vi "NI-USB6001.vi"() -> ()   [LabVIEW 2020]
uses:
  <vilib>/Utility/miscctls.llb/LVPointTypeDef.ctl
  LabVIEW 2020 Toolkits/toolkits_lv2020_32bit/Synchronization.llb/SynchRefs_SetGet.ctl
  LabVIEW 2020 Toolkits/VI Server Toolkit/VI Server Libraries/VI Server_GetControl.llb/VI Server_STR_Get.vi
  LabVIEW 2020 Toolkits/VI Server Toolkit/VI Server Libraries/VI Server_Set Controls.llb/Set STR Control.vi
  LabVIEW 2020 Toolkits/VI Server Toolkit/VI Server Libraries/VI Server_GetControl.llb/VI Server_DBL_Get.vi
  LabVIEW 2020 Toolkits/VI Server Toolkit/VI Server Libraries/VI Server_GetControl.llb/VI Server_Slide_DBL_Get.vi
  LabVIEW 2020 Toolkits/VI Server Toolkit/VI Server Libraries/VI Server_GetControl.llb/VI Server_DAQmx_Device_Get.vi
  LabVIEW 2020 Toolkits/VI Server Toolkit/VI Server Toolkit LV2013.lvlib
panel:
  in  "LastAction.AddToSecuence":bool
  out "System.Message":string="Instrument Initialization Successful." caption="System Message"
  in  "Help":bool
  in  "FP.Hide":bool caption="FrontPanel.Hide"
  in  "EXIT":bool
  in  "Tab.Main":T1(tab)
  in  "AI.Graph.Plots":u16(ring) items=["NI-USB6001/ai0"]
  in  "AI.MultiChannelAcquisition":bool
  in  "AI.PhysicalChannel.Include":bool
  out "AI.ActualSampleRate":dbl=1000.0 caption="Actual Sample Rate" format="%0.2f"
  out "AI.WaveformGraph":waveform(dbl)[](graph) caption="Waveform Graph"
  out "AI.Averaged.Mesurement":dbl caption="Averaged Mesurement" format="%0.4f V"
  in  "AI.Measure":bool
  in  "AI.Number.Of.Samples":i32=100 caption="Number Of Samples"
  in  "AI.SampleRate":dbl=1000.0 caption="Sample Rate" format="%0.0f Hz"
  in  "AI.MinInputLimit":dbl caption="Min Input Limit" min=-10.0 max=10.0 format="%0.3f V"
  in  "AI.MaxInputLimit":dbl caption="Max Input Limit" min=-10.0 max=10.0 format="%0.3f V"
  in  "AI.TerminalConfiguration":u16(ring)=65535 caption="Terminal Configuration" items=["default"=65535, "RSE"=10083, "NRSE"=10078, "Differential"=10106, "Pseudodifferential"=12529]
  in  "AI.Sample.Mode":u16(ring)=12522 caption="Sample Mode" items=["Finite Samples"=10178, "Continuous Samples"=10123]
  in  "AI.Physical.Channel":tag="Dev1/ai0" caption="Physical Channel"
  in  "AO.Update":bool
  out "AO.WaveformGraph":waveform(dbl)(graph) caption="Waveform Graph"
  in  "AO.SampleMode":u16(ring) caption="Sample Mode" items=["Finite Samples"=10178, "Continious Samples"=10123, "Hardware Timed Single Point"=12522]
  in  "AO.OutputVoltage":dbl(slide) caption="Output Voltage" scale=-10.0..10.0 scale format="%0.3f V"
  in  "AO.SinewaveFrequency":dbl=5.0 caption="Sinewave Frequency" min=1e-36 max=5.0 format="%0.2p Hz"
  in  "AO.GenerationMode":u16(ring) caption="Generation Mode" items=["Voltage DC", "Voltage Sine Wave Generation"]
  in  "AO.NumberOfSamples":i32=1000 caption="Number Of Samples" min=2
  in  "AO.SampleRate":dbl=5000.0 caption="Sample Rate" min=1e-07 max=5000.0
  in  "AO.Sample.Clock.Source":tag="OnboardClock" caption="Sample Clock Source"
  out "AO.ActualSampleRate":dbl=1000.0 caption="Actual Sample Rate" format="%0.2f"
  in  "AO.MaxVoltage":dbl=5.0 caption="Max Voltage" format="%0.3f V"
  in  "AO.MinVoltage":dbl=-5.0 caption="Min Voltage" format="%0.3f V"
  in  "AO.Physical.Channel":tag="Dev1/ai0" caption="Physical Channel"
  in  "AO.Output":bool
  out "DO.Port.State.Verify":bool caption="Verified"
  out "DO.Line.State.Verify":bool caption="Verified"
  in  "DO.Line.State":bool caption="State"
  in  "DO.Line":tag="Dev1/port0/line0:7" caption="Line"
  in  "DO.Line.Update":bool caption="Update:"
  in  "DO.Port.Update":bool
  in  "DO.Port.Lines.7:0":u8 caption="Port&Lines 7:0" format="%08b"
  in  "DO.Port":tag="Dev1/port0/line0:7" caption="Port"
  out "DI.Line.State":bool caption="State"
  in  "DI.Port.Update":bool
  out "DI.Port.Lines.0:7":u8 caption="Port&Lines 7:0" format="%08b"
  in  "DI.Port":tag="Dev1/port0/line0:7" caption="Port"
  in  "DI.Line":tag="Dev1/port0/line0:7" caption="Line"
  in  "DI.Line.Update":bool caption="Update:"
  out "ctr0.In.Count":u32 caption="Counts:"
  in  "Cntr.In.Start":bool
  in  "Cntr.In.IntegrationTime":u32=10 format="%.0f msec"
  in  "Cntr.In.Sample.Clock.Source":tag="PFI0" caption="Sample Clock Source"
  in  "Cntr.In.ActiveEdge":u16(ring)=10280 caption="Active Edge" items=["Rising"=10280, "Falling"=10171]
  in  "Cntr.In.Input.Terminal":tag="OnboardClock" caption="Input.Terminal"
  in  "Cntr.In.Channel":tag="Dev1/port0/line0:7" caption="Channel Name"
  in  "TestCase.Execute.All":bool
  in  "TestCase.Execute.Selected":bool
  out "TestCase.SAVE.Success":bool
  in  "TestCase.SAVE":bool
  in  "SequenceFile.Open":bool
  in  "SequenceFile":path caption="Secuence File"
  in  "TestCase.Execute.Step.Pause":bool
  in  "TestCase.Execute.Steps":u16(ring) caption="Test Case: Pause Before Step" items=["1", "2", "3", "4", "5", "6", "7", "8", "9", "10"]
  in  "TestCase.Execute.ABORT":bool
  in  "TestCase.Execute.Next":bool
  in  "TestCase.Execute.Pause":bool
  out "TestCase.ExecutionTime":dbl caption="Execution Time:" format="%0.3f sec"
  in  "TestCase.Execution.StepTime":u32 caption="Seq. Execution: Step Time" format="%d msec"
  in  "TestCaseConfiguration":i32[](listbox) caption="Test Case Configuration"
  in  "TestCase.StepDescription":string caption="Step Description:"
  in  "ProductType":string="USB-6343 (BNC)" caption="Product Type"
  in  "VI.WindowsTitle":string caption="Windows Title"
  in  "DAQmx.Device":tag caption="DAQmx: Device"
  in  "Cont.Measurements.CycleTime":u32 caption="Continius Measurements:\nCycleTime"
  in  "UDP.Test.String2.Send":bool
  in  "UDP.Test.String2":string caption="UDP: Test String 2"
  in  "UDP.Port.BC":u16=58433 caption="UDP: Port.BC"
  in  "UDP.Port.RT":u16=58432 caption="UDP: Port.RT"
  in  "UDP.LocalPort.Write":u16=58434 caption="UDP: Local Port.Write"
  in  "UDP.IP.Address":string="234.5.6.7" caption="UDP: IP Address"
  in  "UDP.Test.String1.Send":bool
  in  "UDP.Test.String1":string caption="UDP: Test String 1"
  in  "UDP.Responce.String.Monitor":bool
  out "UDP.ExecEng.Message.String":string caption="UDP: Execution Engine Message String"
  out "error out":errorcluster={"status"=TRUE, "code"=1055, "source"="Property Node in VI Server Toolkit LV2013.lvlib:VI server_Set Control Value from String Format.vi:5200001->DMM6500_UDP_ExecEng_Instruction_APPLY.vi->DMM6500_UDP_MAIN.vi->Keithley2100.vi"}
  in  "error in":errorcluster
  # "Important Note: Analog Input configuration shall\nstart from Physical Channel selection!"
  # "Digital Input"
  # "Digital Output"
  # "Onboard Clock is not supported as an \nInput Terminal for counter measurements."
  # "Counter Input"
  # "Counter Input"
  # "M"
  # "Multicast IP addresses must be in the 224.0.0.0 to 239.255.255.255 range."
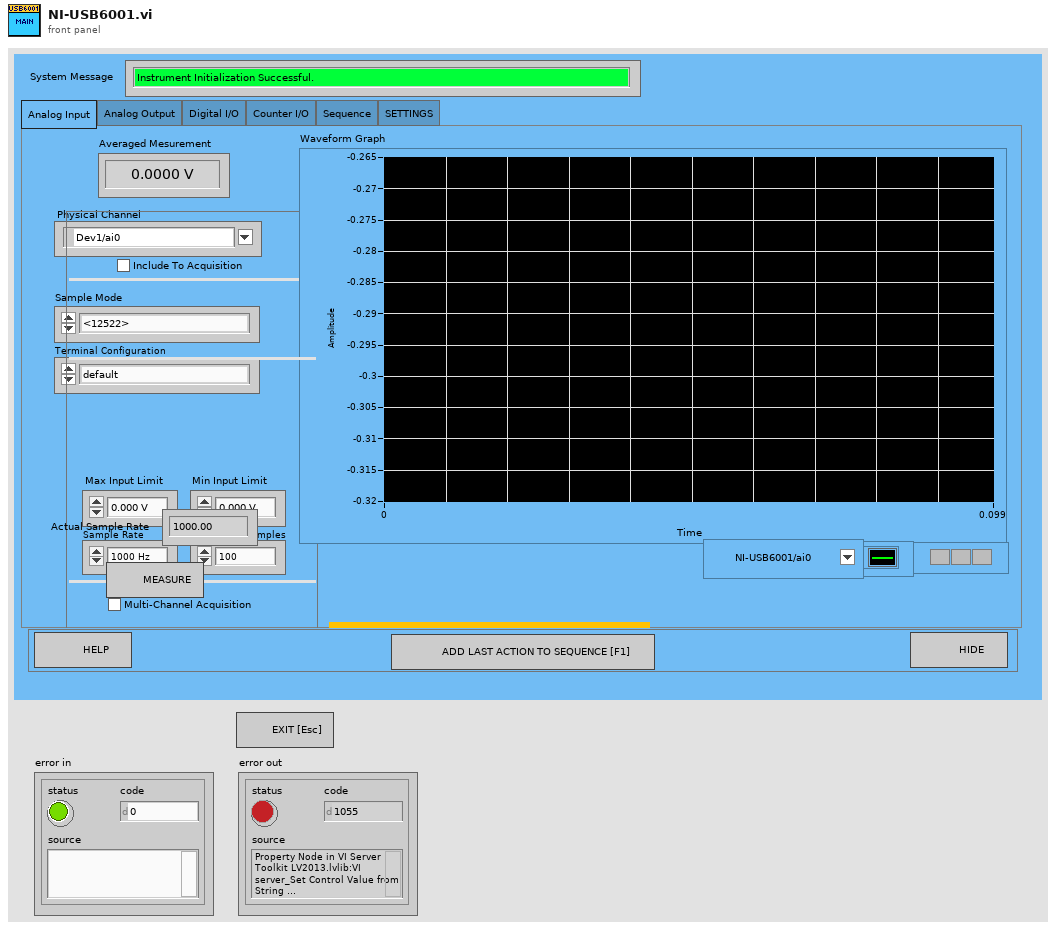
[diagram p1: front panel]
types:
  T1 = enum32{"Analog Input", "Analog Output", "Digital I/O", "Counter I/O", "Sequence", "SETTINGS"}
  T2 = typedef "LVPointTypeDef.ctl" = cluster{"Horizontal":i16, "Vertical":i16}
  T3 = typedef "VI Server_RefsCluster.ctl" = cluster{"Labels":string[], "Refs":refnum<vi>[], "VI Ref":refnum<vi>}
  T4 = typedef "SynchRefs_SetGet.ctl" = enum16{"Set", "Get"}
  T5 = cluster{"Color":u32, "PointStyle":u8, "LineStyle":u8, "Interp":u8, "LineWidth":u8, "BarPlotStyle":u8, "FillTo":i16, "XScaleIdx":u32, "YScaleIdx":u32, "Anti-Aliased":bool, "LabelFormat":u8, "TransitionType":u8, "TransitionLocation":u8, "DigitalLineStyle":u8}
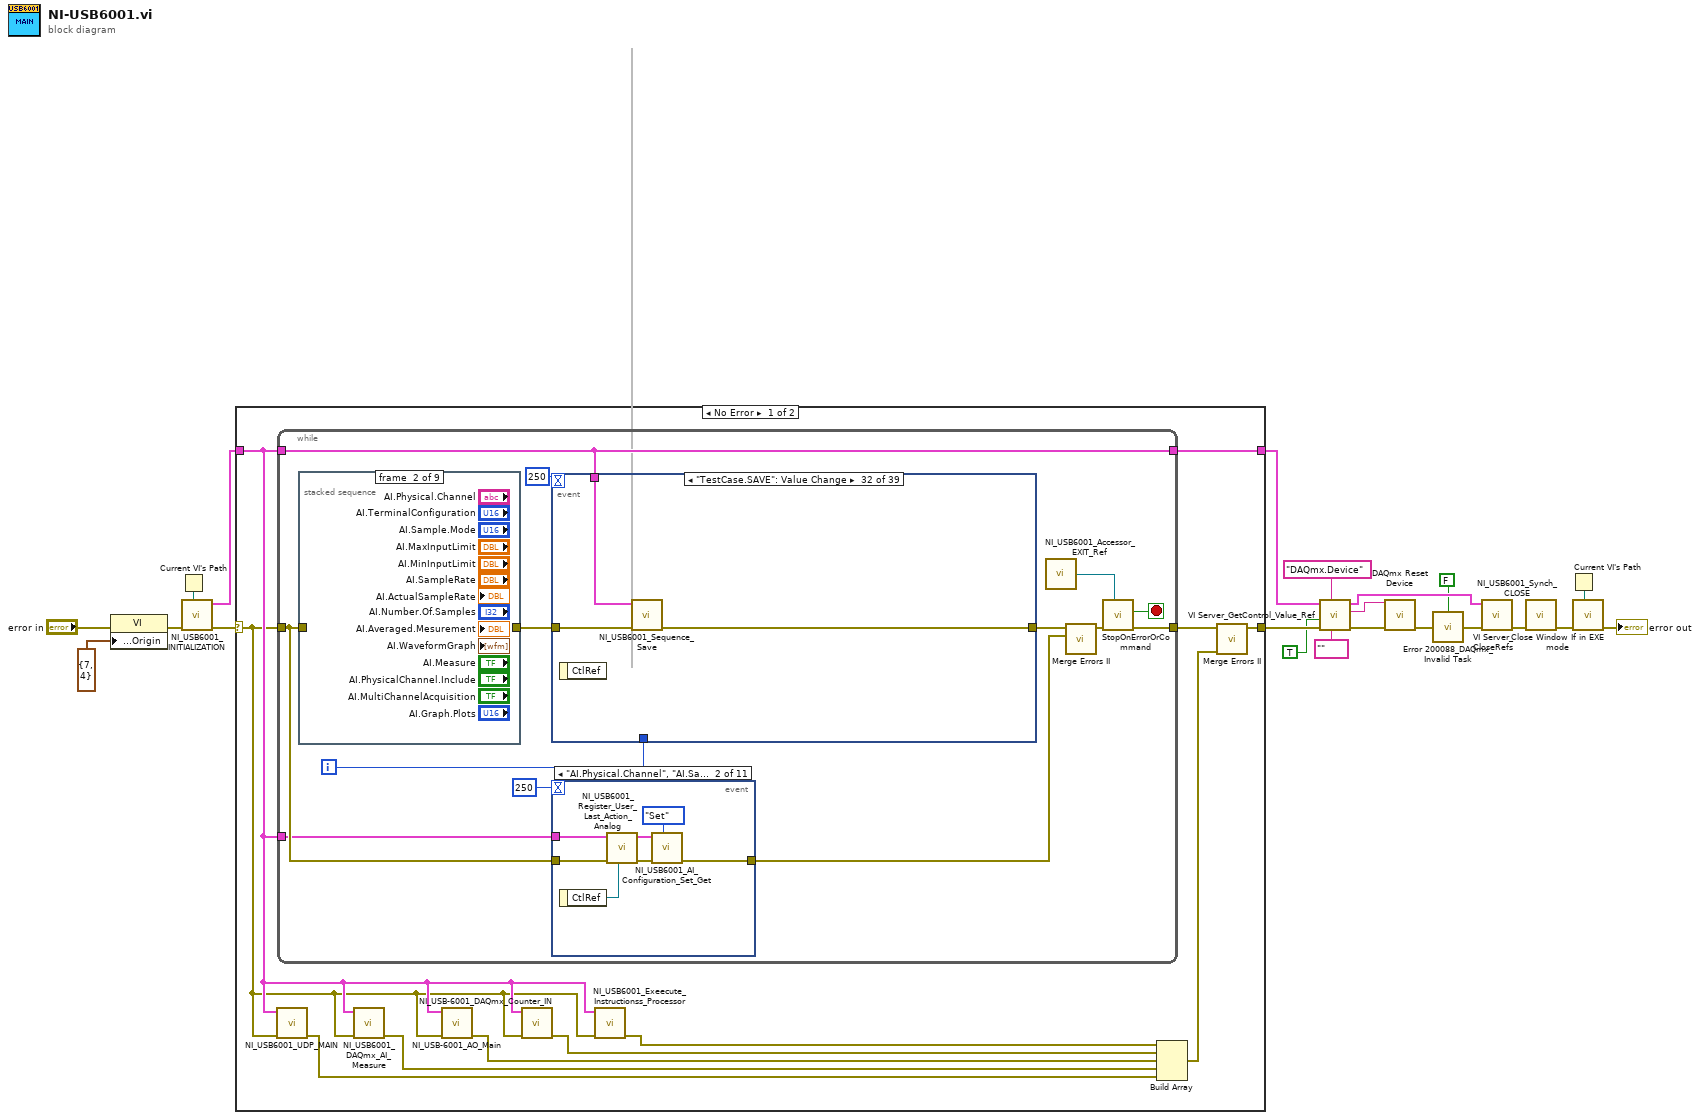
[diagram p0: block diagram]
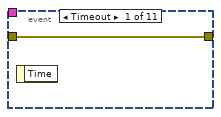
[diagram p2: hidden frame]
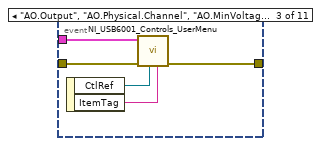
[diagram p3: hidden frame]
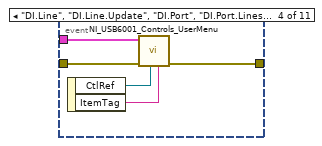
[diagram p4: hidden frame]
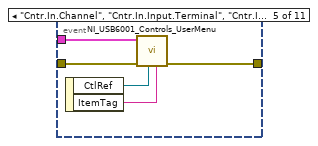
[diagram p5: hidden frame]
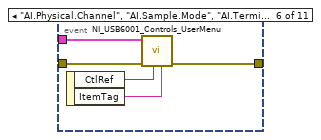
[diagram p6: hidden frame]
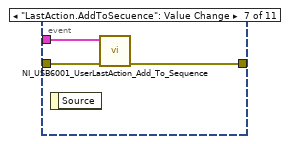
[diagram p7: hidden frame]
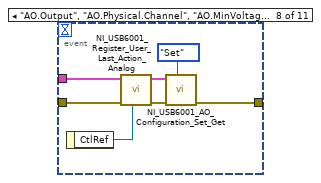
[diagram p8: hidden frame]
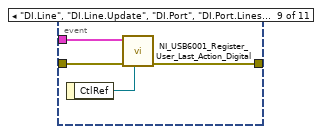
[diagram p9: hidden frame]
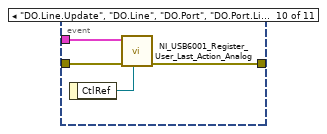
[diagram p10: hidden frame]
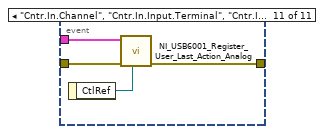
[diagram p11: hidden frame]
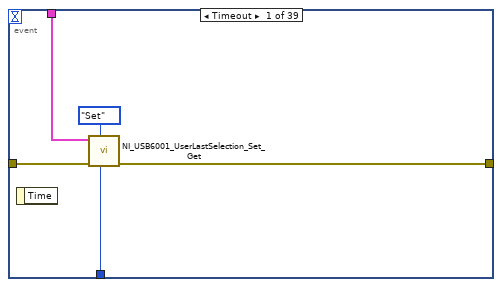
[diagram p12: hidden frame]
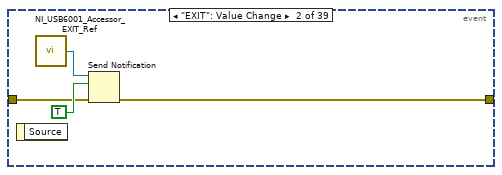
[diagram p13: hidden frame]
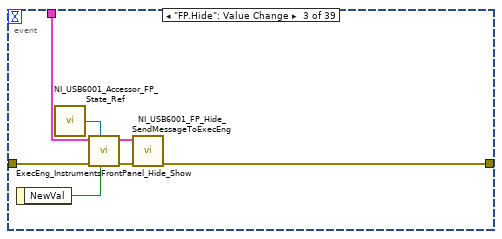
[diagram p14: hidden frame]
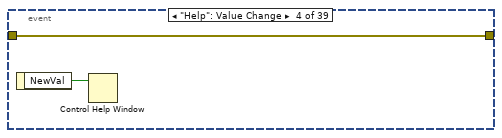
[diagram p15: hidden frame]
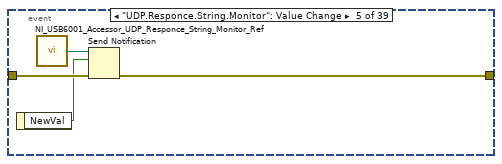
[diagram p16: hidden frame]
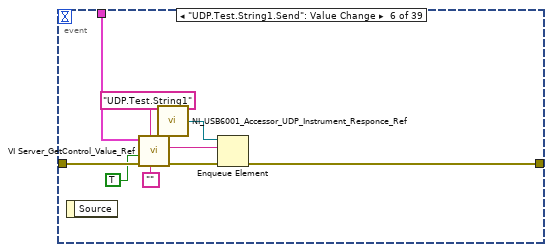
[diagram p17: hidden frame]
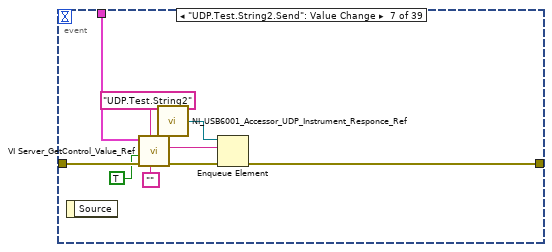
[diagram p18: hidden frame]
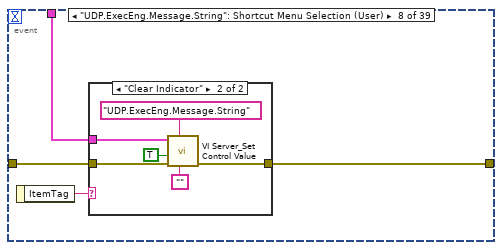
[diagram p19: hidden frame]
diagram:
  n1 = property class="VI"(error in="error in", "Front Panel Window:Origin"=T2 {"Horizontal"=7, "Vertical"=4}) -> (error out=w21:errorcluster)  [unwired: 1 in, 1 out]
  n2 = Current VI's Path() -> (path=w1:path)
  n3 = call "NI_USB6001_INITIALIZATION.vi"("Top VI Path"=w1, "error in (no error)"=w21) -> ("error out"=w20:errorcluster, "VI Server Cluster.OUT"=w19:T3)  [unwired: 8 in]
  n4 = case shown="No Error" w20 {
    selector: w20 -> [w23 w321]
    tunnel: [w29 w321] -> w12
    tunnel: w19 -> [w24 w320]
    tunnel: [w32 w320] -> w10
    frame No Error {
      n5 = call "NI_USB6001_UDP_MAIN.vi"("error in (no error)"=w23, "VI Server.RefsCluster"=w24) -> ("error out"=w31:errorcluster)  [unwired: 9 in]
      n6 = while {
        tunnel: w23 -> [w37]
        tunnel: [w41] -> w30
        tunnel: w24 -> [w42]
        tunnel: [w42] -> w32
        tunnel: w24 -> [w36]
        i -> [w43]
        stop <- w40 stop-if-true
        n7 = stacked-sequence {
          tunnel: w37 -> [w319 _ _ _ _ _ _ _ _]
          tunnel: [w319 _ _ _ _ _ _ _ _] -> w45
          frame #0 {
          }
          frame #1 {
          }
          frame #2 {
          }
          frame #3 {
          }
          frame #4 {
          }
          frame #5 {
          }
          frame #6 {
          }
          frame #7 {
          }
          frame #8 {
          }
        }
        n8 = event shown="[31] \"TestCase.SAVE\": Value Change" {
          selector: _ -> [_ _ _ _ _ _ _ _ _ _ _ _ _ _ _ _ _ _ _ _ _ _ _ _ _ _ _ _ _ _ _ _ _ _ _ _ _ _ _]
          dyn-events: _ -> [_ _ _ _ _ _ _ _ _ _ _ _ _ _ _ _ _ _ _ _ _ _ _ _ _ _ _ _ _ _ _ _ _ _ _ _ _ _ _]
          timeout: 250 -> [_ _ _ _ _ _ _ _ _ _ _ _ _ _ _ _ _ _ _ _ _ _ _ _ _ _ _ _ _ _ _ _ _ _ _ _ _ _ _]
          tunnel: w45 -> [w99 w101 w110 w113 w117 w126 w135 w139 w152 w158 w171 w174 w175 w180 w183 w190 w194 w198 w204 w212 w237 w240 w244 w247 w250 w253 w257 w266 w274 w277 w282 w285 w288 w291 w294 w298 w310 w312 w316]
          tunnel: w43 -> [w98 _ _ _ _ _ _ _ _ _ _ _ _ _ _ _ _ _ _ _ _ _ _ _ _ _ _ _ _ _ _ _ _ _ _ _ _ _ _]
          tunnel: [w96 w103 w111 w113 w115 w124 w133 w137 w149 w154 w163 w172 w175 w176 w182 w186 w191 w197 w203 w206 w225 w239 w242 w245 w248 w252 w255 w263 w272 w278 w280 w283 w286 w289 w292 w297 w309 w314 w315] -> w35
          tunnel: w42 -> [w97 _ w107 _ _ w123 w132 w136 w151 w157 w170 w173 _ w179 w181 w189 w193 _ _ w211 w235 w238 w243 w246 w249 w254 w256 _ w273 w276 w281 w284 w287 w290 w293 w296 _ _ _]
          event Timeout {
            n9 = event-data() -> ()  [unwired: 1 in, 1 out]
            n10 = call "NI_USB6001_UserLastSelection_Set_Get.vi"("LoopCounter"=w98, "SynchRefs.Set/Get"=SynchRefs_SetGet."Set", "error in"=w99, "VI Server.RefsCluster"=w97) -> ("error out"=w96:errorcluster)  [unwired: 6 in, 1 out]
          }
          event "EXIT": Value Change {
            n11 = event-data() -> ()  [unwired: 1 in, 1 out]
            n12 = call "NI_USB6001_Accessor_EXIT_Ref.vi"() -> ("EXIT"=w104:refnum<notifier>)  [unwired: 6 in]
            n13 = Send Notification(notification=TRUE, notifier=w104, error in (no error)=w101) -> (error out=w103:errorcluster)  [unwired: 1 out]
          }
          event "FP.Hide": Value Change {
            n14 = event-data() -> ("NewVal"=w108:bool)  [unwired: 1 in]
            n15 = call "NI_USB6001_Accessor_FP_State_Ref.vi"() -> ("FP.State"=w105:refnum<notifier>)  [unwired: 6 in]
            n16 = call "ExecEng_InstrumentsFrontPanel_Hide_Show.vi"("FP.Hide/Show"=w108, "FP.State"=w105, "error in (no error)"=w110, "VI Server Cluster"=w107) -> ("error out"=w109:errorcluster, "VI Server Cluster DUP"=w106:T3)  [unwired: 6 in]
            n17 = call "NI_USB6001_FP_Hide_SendMessageToExecEng.vi"("error in (no error)"=w109, "VI Server Cluster"=w106) -> ("error out"=w111:errorcluster)  [unwired: 9 in]
          }
          event "Help": Value Change {
            n18 = event-data() -> ("NewVal"=w112:bool)  [unwired: 1 in]
            n19 = Control Help Window(1:w112) -> ()  [unwired: 1 in]
          }
          event "UDP.Responce.String.Monitor": Value Change {
            n20 = event-data() -> ("NewVal"=w114:bool)  [unwired: 1 in]
            n21 = call "NI_USB6001_Accessor_UDP_Responce_String_Monitor_Ref.vi"() -> ("UDP.ExecEng.Command.String.Monitor"=w116:refnum<notifier>)  [unwired: 6 in]
            n22 = Send Notification(notification=w114, notifier=w116, error in (no error)=w117) -> (error out=w115:errorcluster)  [unwired: 1 out]
          }
          event "UDP.Test.String1.Send": Value Change {
            n23 = event-data() -> ()  [unwired: 1 in, 1 out]
            n24 = call-poly "VI Server_GetControl_Value_Ref.vi"("DataType"="", "Control.Label"="UDP.Test.String1", "error in"=w126, "SingleInstance"=TRUE, "VI Server.RefsCluster"=w123) -> ("error out"=w125:errorcluster, "Value"=w118:string)  [unwired: 3 in, 2 out]
            n25 = call "NI_USB6001_Accessor_UDP_Instrument_Responce_Ref.vi"() -> ("UDP.Instrument.Responce.Q"=w119:refnum<queue>)  [unwired: 6 in]
            n26 = Enqueue Element(queue=w119, element=w118, error in (no error)=w125) -> (error out=w124:errorcluster)  [unwired: 1 in, 2 out]
          }
          event "UDP.Test.String2.Send": Value Change {
            n27 = event-data() -> ()  [unwired: 1 in, 1 out]
            n28 = call-poly "VI Server_GetControl_Value_Ref.vi"("DataType"="", "Control.Label"="UDP.Test.String2", "error in"=w135, "SingleInstance"=TRUE, "VI Server.RefsCluster"=w132) -> ("error out"=w134:errorcluster, "Value"=w127:string)  [unwired: 3 in, 2 out]
            n29 = call "NI_USB6001_Accessor_UDP_Instrument_Responce_Ref.vi"() -> ("UDP.Instrument.Responce.Q"=w128:refnum<queue>)  [unwired: 6 in]
            n30 = Enqueue Element(queue=w128, element=w127, error in (no error)=w134) -> (error out=w133:errorcluster)  [unwired: 1 in, 2 out]
          }
          event "UDP.ExecEng.Message.String": Shortcut Menu Selection (User) {
            n31 = event-data() -> ("ItemTag"=w138:string)  [unwired: 1 in]
            n32 = case shown="\"Clear Indicator\"" w138 {
              tunnel: w139 -> [w140 w146]
              tunnel: [w140 w145] -> w137
              tunnel: w136 -> [_ w144]
              frame "", Default {
              }
              frame "Clear Indicator" {
                n33 = call-poly "VI Server_Set Control Value.vi"("New Value"="", "Label"="UDP.ExecEng.Message.String" ("Control.Label"), "error in"=w146, "Single Instance (T)"=TRUE ("SingleInstance"), "VI Server Cluster"=w144) -> ("error out"=w145:errorcluster)  [unwired: 4 in, 2 out]
              }
            }
          }
          event "DAQmx.Device": Value Change {
            n34 = event-data() -> ("NewVal"=w148:tag)  [unwired: 1 in]
            n35 = call "NI_USB6001_DAQmx_LimitPhysicalChannelsToDevice.vi"("error in (no error)"=w152, "VI Server Cluster"=w151) -> ("error out"=w150:errorcluster, "VI Server Cluster.DUP"=w147:T3)  [unwired: 7 in, 1 out]
            n36 = call "NI_USB6001_DAQmx_DeviceName_Changed_UpdateSet_Get_Sections.vi"("DAQmx.Device"=w148, "error in (no error)"=w150, "VI Server Cluster"=w147) -> ("error out"=w149:errorcluster)  [unwired: 8 in]
          }
          event "AI.Physical.Channel": Value Change {
            n37 = event-data() -> ()  [unwired: 1 in, 1 out]
            n38 = call "NI_USB6001_AI_Configuration_Set_Get.vi"("SynchRefs.Set/Get"=SynchRefs_SetGet."Get", "error in (no error)"=w158, "VI Server Cluster"=w157) -> ("error out"=w153:errorcluster, "VI Server Cluster.DUP"=w155:T3)  [unwired: 6 in, 1 out]
            n39 = call "NI_USB6001_AI_Graph_PopulatePlotSelector.vi"("error in (no error)"=w153, "VI Server Cluster"=w155) -> ("error out"=w154:errorcluster)  [unwired: 9 in]
          }
          event "TestCaseConfiguration": Value Change {
            n40 = event-data() -> ()  [unwired: 1 in, 1 out]
            n41 = call "VI Server_M_ClmnListBox_1orMoreSelection_ItemNames_GET.vi"("Label"="TestCaseConfiguration", "error in"=w171, "SingleInstance"=TRUE, "VI Server.RefsCluster"=w170) -> ("error out"=w165:errorcluster, "Item Names"=w167:string[][], "VI Server.RefsCluster.DUP"=w164:T3, "Value"=w166:i32[])  [unwired: 1 in, 3 out]
            n42 = Index Array(array=w166) -> (element=w159:i32)  [unwired: 1 in]
            n43 = Index Array(array=w167, index (row)=w159, index (col)=0 ("index (row)")) -> (element=w160:string)
            n44 = call "VI Server_Set Text Ring by Item Selected_SignalingValue.vi"("Label"="TestCase.Execute.Steps" ("Control.Label"), "error in"=w165, "Item"=w160, "VI Server Cluster"=w164) -> ("error out"=w163:errorcluster)  [unwired: 5 in, 2 out]
          }
          event "AI.MultiChannelAcquisition": Value Change {
            n45 = event-data() -> ()  [unwired: 1 in, 1 out]
            n46 = call "NI_USB6001_AI_MultiChannelACQ_UpdateGraph_Plots.vi"("error in (no error)"=w174, "VI Server Cluster"=w173) -> ("error out"=w172:errorcluster)  [unwired: 9 in]
          }
          event "AI.Measure": Value Change {
            n47 = event-data() -> ()  [unwired: 1 in, 1 out]
          }
          event "AI.WaveformGraph": Plot Attribute Change {
            n48 = event-data() -> ("OldAttrib"=w178:T5, "NewAttrib"=w177:T5)  [unwired: 1 in]
            n49 = call "NI_USB6001_AI_Graph_PlotAttribute_ValueChanged.vi"("NewAttrib"=w177, "OldAttrib"=w178, "error in (no error)"=w180, "VI Server Cluster"=w179) -> ("error out"=w176:errorcluster)  [unwired: 7 in]
          }
          event "AO.Physical.Channel": Value Change {
            n50 = event-data() -> ()  [unwired: 1 in, 1 out]
            n51 = call "NI_USB6001_AO_Configuration_Set_Get.vi"("error in (no error)"=w183, "VI Server Cluster"=w181) -> ("error out"=w182:errorcluster)  [unwired: 7 in, 2 out]
          }
          event "AO.GenerationMode": Value Change {
            n52 = event-data() -> ("NewVal"=w184:u16)  [unwired: 1 in]
            n53 = call "NI_USB6001_AO_GenerationMode.vi"("AO.GenerationMode"=w184, "error in (no error)"=w190, "VI Server Cluster"=w189) -> ("error out"=w187:errorcluster)  [unwired: 7 in, 1 out]
            n54 = call "NI_USB-6001_Accessor_ao_Waveform_Array_Update_Ref.vi"() -> ("ao.Waveform.Array.Update"=w185:refnum<notifier>)  [unwired: 6 in]
            n55 = Send Notification(notification=TRUE, notifier=w185, error in (no error)=w187) -> (error out=w186:errorcluster)  [unwired: 1 out]
          }
          event "AO.OutputVoltage", "AO.SinewaveFrequency": Value Change {
            n56 = event-data() -> ()  [unwired: 1 in, 1 out]
            n57 = call "VI Server_CycleEventBySignalingValue.vi"("Label"="AO.GenerationMode", "error in"=w194, "VI Server.RefsCluster"=w193) -> ("error out"=w191:errorcluster)  [unwired: 7 in, 1 out]
          }
          event "AO.Output": Value Change {
            n58 = event-data() -> ("NewVal"=w196:bool)  [unwired: 1 in]
            n59 = call "NI_USB-6001_Accessor_ao0_State_Ref.vi"() -> ("ao0.State"=w199:refnum<notifier>)  [unwired: 6 in]
            n60 = Send Notification(notification=w196, notifier=w199, error in (no error)=w198) -> (error out=w201:errorcluster)  [unwired: 1 out]
            n61 = call "NI_USB-6001_Accessor_ao_Waveform_Array_Update_Ref.vi"() -> ("ao.Waveform.Array.Update"=w200:refnum<notifier>)  [unwired: 6 in]
            n62 = Send Notification(notification=TRUE, notifier=w200, error in (no error)=w201) -> (error out=w197:errorcluster)  [unwired: 1 out]
          }
          event "AO.Update": Value Change {
            n63 = event-data() -> ()  [unwired: 1 in, 1 out]
            n64 = call "NI_USB-6001_Accessor_ao_Waveform_Array_Update_Ref.vi"() -> ("ao.Waveform.Array.Update"=w205:refnum<notifier>)  [unwired: 6 in]
            n65 = Send Notification(notification=TRUE, notifier=w205, error in (no error)=w204) -> (error out=w203:errorcluster)  [unwired: 1 out]
          }
          event "AO.Sample.Clock.Source", "AO.SampleMode", "AO.SampleRate", "AO.NumberOfSamples": Value Change {
            n66 = event-data() -> ()  [unwired: 1 in, 1 out]
            n67 = call "NI_USB-6001_Accessor_ao0_State_Ref.vi"() -> ("ao0.State"=w209:refnum<notifier>)  [unwired: 6 in]
            n68 = call "NI_USB6001_AO_ConfigurationAtributes.vi"("error in (no error)"=w212, "VI Server Cluster"=w211) -> ("error out"=w207:errorcluster)  [unwired: 8 in, 1 out]
            n69 = Get Notifier Status(notifier=w209, error in (no error)=w207) -> (current notification=w210:bool, error out=w208:errorcluster)  [unwired: 3 out]
            n70 = case shown="True" w210 {
              tunnel: [w213 w218] -> w206
              tunnel: w208 -> [w213 w215]
              tunnel: w209 -> [_ w214]
              frame False {
              }
              frame True {
                w217 = TRUE ("notification")
                n71 = Send Notification(notification=FALSE, notifier=w214, error in (no error)=w215) -> (error out=w220:errorcluster)  [unwired: 1 out]
                n72 = call "NI_USB-6001_Accessor_ao_Waveform_Array_Update_Ref.vi"() -> ("ao.Waveform.Array.Update"=w221:refnum<notifier>)  [unwired: 6 in]
                n73 = Send Notification(notification=w217, notifier=w221, error in (no error)=w220) -> (error out=w219:errorcluster)  [unwired: 1 out]
                n74 = Send Notification(notification=w217, notifier=w214, error in (no error)=w219) -> (error out=w218:errorcluster)  [unwired: 1 out]
              }
            }
          }
          event "AO.MaxVoltage", "AO.MinVoltage": Value Change {
            w228 = 0.0
            w227 = TRUE ("SingleInstance")
            n75 = event-data() -> ()  [unwired: 1 in, 1 out]
            n76 = call-poly "VI Server_GetControl_Value_Ref.vi"("DataType"=w228, "Control.Label"="AO.MaxVoltage", "error in"=w237, "SingleInstance"=w227, "VI Server.RefsCluster"=w235) -> ("error out"=w236:errorcluster, "Value"=w222:dbl, "VI Server.RefsCluster.DUP"=w234:T3)  [unwired: 3 in, 1 out]
            n77 = call-poly "VI Server_GetControl_Value_Ref.vi"("DataType"=w228, "Control.Label"="AO.MinVoltage", "error in"=w236, "SingleInstance"=w227, "VI Server.RefsCluster"=w234) -> ("error out"=w231:errorcluster, "Value"=w223:dbl, "VI Server.RefsCluster.DUP"=w230:T3)  [unwired: 3 in, 1 out]
            n78 = call-poly "VI Server_GetControl_Value_Ref.vi"("DataType"=w228, "Control.Label"="AO.OutputVoltage", "error in"=w231, "SingleInstance"=w227, "VI Server.RefsCluster"=w230) -> ("error out"=w226:errorcluster, "Control.Ref"=w224:refnum<vi>)  [unwired: 3 in, 2 out]
            n79 = property class="Slide (strict)"(reference=w224, error in=w226, "Scale.Minimum"=w223, "Scale.Maximum"=w222) -> (error out=w225:errorcluster)  [unwired: 1 out]
          }
          event "DI.Line.Update": Value Change {
            n80 = event-data() -> ()  [unwired: 1 in, 1 out]
            n81 = call "NI_USB6001_Digital_Input_Line_Update.vi"("error in (no error)"=w240, "VI Server Cluster"=w238) -> ("error out"=w239:errorcluster)  [unwired: 9 in]
          }
          event "DI.Port": Value Change {
            n82 = event-data() -> ("NewVal"=w241:tag)  [unwired: 1 in]
            n83 = call "NI_USB6001_DI_Port_ValueChanged.vi"("DI.Port"=w241, "error in (no error)"=w244, "VI Server Cluster"=w243) -> ("error out"=w242:errorcluster)  [unwired: 8 in]
          }
          event "DI.Port.Update": Value Change {
            n84 = event-data() -> ()  [unwired: 1 in, 1 out]
            n85 = call "NI_USB6001_DI_Port_Update.vi"("error in (no error)"=w247, "VI Server Cluster"=w246) -> ("error out"=w245:errorcluster)  [unwired: 9 in]
          }
          event "DO.Line.Update": Value Change {
            n86 = event-data() -> ()  [unwired: 1 in, 1 out]
            n87 = call "NI_USB6001_Digital_Output_Line_Update.vi"("error in (no error)"=w250, "VI Server Cluster"=w249) -> ("error out"=w248:errorcluster)  [unwired: 9 in]
          }
          event "DO.Port": Value Change {
            n88 = event-data() -> ("NewVal"=w251:tag)  [unwired: 1 in]
            n89 = call "NI_USB6001_D0_Port_ValueChanged_v2.vi"("DI.Port"=w251, "error in (no error)"=w253, "VI Server Cluster"=w254) -> ("error out"=w252:errorcluster)  [unwired: 8 in]
          }
          event "DO.Port.Update": Value Change {
            n90 = event-data() -> ()  [unwired: 1 in, 1 out]
            n91 = call "NI_USB6001_DO_Port_Update.vi"("error in (no error)"=w257, "VI Server Cluster"=w256) -> ("error out"=w255:errorcluster)  [unwired: 9 in]
          }
          event "DO.Port.Lines.7:0", "DI.Port.Lines.0:7": Mouse Down {
            n92 = event-data() -> ("CtlRef"=w265:refnum<vi>)  [unwired: 1 in]
            n93 = property class="DigNum (strict)"(reference=w265, error in=w266) -> (reference out=w262:refnum<vi>, error out=w264:errorcluster, "FormatString"=w259:string)
            n94 = Match Pattern(string=w259, regular expression="[0-9]+") -> (after substring=w258:string)  [unwired: 1 in, 3 out]
            n95 = case shown="\"b\", Default" w258 {
              tunnel: ["%.0f" "%02x" "%02o" "%08b"] -> w261
              frame "f" {
              }
              frame "x" {
              }
              frame "o" {
              }
              frame "b", Default {
              }
            }
            n96 = property class="DigNum (strict)"(reference=w262, error in=w264, "FormatString"=w261) -> (error out=w263:errorcluster)  [unwired: 1 out]
          }
          event "Cntr.In.Channel": Value Change {
            n97 = event-data() -> ("NewVal"=w271:tag)  [unwired: 1 in]
            n98 = call "NI-USB6001_Counter_IN_GetStateFromFile.vi"("Counter.IN.Channel"=w271, "error in (no error)"=w274, "VI Server Cluster"=w273) -> ("error out"=w272:errorcluster)  [unwired: 7 in, 1 out]
          }
          event "Cntr.In.Start": Value Change {
            n99 = event-data() -> ("NewVal"=w275:bool)  [unwired: 1 in]
            n100 = call "NI-USB6001_Counter_IN_SaveStateToFile.vi"("Cntr.In.Start"=w275, "error in (no error)"=w277, "VI Server Cluster"=w276) -> ("error out"=w278:errorcluster)  [unwired: 7 in, 1 out]
          }
          event "TestCaseConfiguration": Shortcut Menu Selection (User) {
            n101 = event-data() -> ("ItemTag"=w279:string)  [unwired: 1 in]
            n102 = call "NI_USB6001_Sequence_TestCaseConfig_UserMenu.vi"("ItemTag"=w279, "error in (no error)"=w282, "VI Server.RefsCluster"=w281) -> ("error out"=w280:errorcluster)  [unwired: 8 in]
          }
          event "TestCase.SAVE": Value Change {
            n103 = event-data() -> ()  [unwired: 1 in, 1 out]
            n104 = call "NI_USB6001_Sequence_Save.vi"("error in (no error)"=w285, "VI Server Cluster"=w284) -> ("error out"=w283:errorcluster)  [unwired: 9 in]
          }
          event "SequenceFile.Open": Value Change {
            n105 = event-data() -> ()  [unwired: 1 in, 1 out]
            n106 = call "NI_USB6001_Sequence_Open.vi"("error in (no error)"=w288, "VI Server Cluster"=w287) -> ("error out"=w286:errorcluster)  [unwired: 9 in]
          }
          event "TestCase.Execute.Selected": Value Change {
            n107 = event-data() -> ()  [unwired: 1 in, 1 out]
            n108 = call "NI_USB6001_ExecuteSelectedInstruction.vi"("error in (no error)"=w291, "VI Server Cluster"=w290) -> ("error out"=w289:errorcluster)  [unwired: 9 in]
          }
          event "TestCase.Execute.All": Value Change {
            n109 = event-data() -> ()  [unwired: 1 in, 1 out]
            n110 = call "NI_USB6001_Execute_All_Instruction.vi"("error in (no error)"=w294, "VI Server Cluster"=w293) -> ("error out"=w292:errorcluster)  [unwired: 9 in]
          }
          event "LastAction.AddToSecuence": Value Change {
            w306 = "TestCaseConfiguration" ("Label")
            w305 = TRUE ("SingleInstance")
            n111 = event-data() -> ()  [unwired: 1 in, 1 out]
            n112 = call "NI_USB6001_Accessor_RegisteredUserEvent_Ref.vi"() -> ("RegisteredUserEvent"=w295:refnum<notifier>)  [unwired: 6 in]
            n113 = Get Notifier Status(notifier=w295, error in (no error)=w298) -> (current notification=w301:string[], error out=w299:errorcluster)  [unwired: 3 out]
            n114 = call "VI Server_M_ClmnListBox_1orMoreSelection_ItemNames_GET.vi"("Label"=w306, "error in"=w299, "SingleInstance"=w305, "VI Server.RefsCluster"=w296) -> ("error out"=w302:errorcluster, "Item Names"=w300:string[][], "VI Server.RefsCluster.DUP"=w303:T3)  [unwired: 1 in, 4 out]
            n115 = Build Array (concatenate)(w300, w301) -> (w304:string[][])
            n116 = call "VI Server_M_ClmnListBox_ItemNames_SET.vi"("Item Names"=w304, "Label"=w306, "error in"=w302, "SingleInstance"=w305, "VI Server.RefsCluster"=w303) -> ("error out"=w297:errorcluster)  [unwired: 4 in, 2 out]
          }
          event "TestCase.Execute.Pause": Value Change {
            n117 = event-data() -> ("NewVal"=w308:bool)  [unwired: 1 in]
            n118 = call "NI_USB6001_TestCase_Execution_Pause_Ref.vi"() -> ("SequenceExecution.StepPAUSE"=w307:refnum<notifier>)  [unwired: 6 in]
            n119 = Send Notification(notification=w308, notifier=w307, error in (no error)=w310) -> (error out=w309:errorcluster)  [unwired: 1 out]
          }
          event "TestCase.Execute.Next": Value Change {
            n120 = event-data() -> ()  [unwired: 1 in, 1 out]
            n121 = call "NI_USB6001_TestCase_Execution_NEXT_Ref.vi"() -> ("SequenceExecution.StepNEXT"=w311:refnum<notifier>)  [unwired: 6 in]
            n122 = Send Notification(notification=TRUE, notifier=w311, error in (no error)=w312) -> (error out=w314:errorcluster)  [unwired: 1 out]
          }
          event "TestCase.Execute.ABORT": Value Change {
            n123 = event-data() -> ()  [unwired: 1 in, 1 out]
            n124 = call "NI_USB6001_Accessor_Sequence_Execution_ABORT_Ref.vi"() -> ("SequenceExecution.ABORT"=w317:refnum<notifier>)  [unwired: 6 in]
            n125 = Send Notification(notification=TRUE, notifier=w317, error in (no error)=w316) -> (error out=w315:errorcluster)  [unwired: 1 out]
          }
        }
        n126 = event shown="[1] \"AI.Physical.Channel\", \"AI.Sample.Mode\", \"AI.TerminalConfiguration\", \"AI.MaxInputLimit\", \"AI.MinInputLimit\", \"AI.SampleRate\", \"AI.Number.Of.Samples\", \"AI.PhysicalChannel.Include\", \"AI.MultiChannelAcquisition\", \"AI.Measure\": Value Change" {
          selector: _ -> [_ _ _ _ _ _ _ _ _ _ _]
          dyn-events: _ -> [_ _ _ _ _ _ _ _ _ _ _]
          timeout: 250 -> [_ _ _ _ _ _ _ _ _ _ _]
          tunnel: w37 -> [w46 w50 w57 w62 w67 w73 w76 w83 w87 w91 w95]
          tunnel: [w46 w53 w56 w61 w66 w72 w74 w78 w85 w90 w94] -> w33
          tunnel: w36 -> [_ w51 w58 w63 w68 w71 w75 w82 w86 w89 w93]
          event Timeout {
            n127 = event-data() -> ()  [unwired: 1 in, 1 out]
          }
          event "AI.Physical.Channel", "AI.Sample.Mode", "AI.TerminalConfiguration", "AI.MaxInputLimit", "AI.MinInputLimit", "AI.SampleRate", "AI.Number.Of.Samples", "AI.PhysicalChannel.Include", "AI.MultiChannelAcquisition", "AI.Measure": Value Change {
            n128 = event-data() -> ("CtlRef"=w48:refnum<vi>)  [unwired: 1 in]
            n129 = call "NI_USB6001_Register_User_Last_Action_Analog.vi"("Control in"=w48, "error in (no error)"=w50, "VI Server Cluster"=w51) -> ("error out"=w49:errorcluster, "VI Server Cluster.DUP"=w47:T3)  [unwired: 7 in]
            n130 = call "NI_USB6001_AI_Configuration_Set_Get.vi"("SynchRefs.Set/Get"=SynchRefs_SetGet."Set", "error in (no error)"=w49, "VI Server Cluster"=w47) -> ("error out"=w53:errorcluster)  [unwired: 6 in, 2 out]
          }
          event "AO.Output", "AO.Physical.Channel", "AO.MinVoltage", "AO.MaxVoltage", "AO.ActualSampleRate", "AO.Sample.Clock.Source", "AO.SampleRate", "AO.NumberOfSamples", "AO.GenerationMode", "AO.SinewaveFrequency", "AO.OutputVoltage", "AO.SampleMode", "AO.Update": Shortcut Menu Selection (User) {
            n131 = event-data() -> ("CtlRef"=w55:refnum<vi>, "ItemTag"=w54:string)  [unwired: 1 in]
            n132 = call "NI_USB6001_Controls_UserMenu.vi"("ItemTag"=w54, "Control Ref"=w55, "error in (no error)"=w57, "VI Server Cluster"=w58) -> ("error out"=w56:errorcluster)  [unwired: 7 in]
          }
          event "DI.Line", "DI.Line.Update", "DI.Port", "DI.Port.Lines.0:7", "DI.Port.Update", "DO.Line.Update", "DO.Line", "DO.Port", "DO.Port.Lines.7:0", "DO.Port.Update", "DO.Line.State": Shortcut Menu Selection (User) {
            n133 = event-data() -> ("CtlRef"=w60:refnum<vi>, "ItemTag"=w59:string)  [unwired: 1 in]
            n134 = call "NI_USB6001_Controls_UserMenu.vi"("ItemTag"=w59, "Control Ref"=w60, "error in (no error)"=w62, "VI Server Cluster"=w63) -> ("error out"=w61:errorcluster)  [unwired: 7 in]
          }
          event "Cntr.In.Channel", "Cntr.In.Input.Terminal", "Cntr.In.ActiveEdge", "Cntr.In.Sample.Clock.Source", "Cntr.In.IntegrationTime", "Cntr.In.Start": Shortcut Menu Selection (User) {
            n135 = event-data() -> ("CtlRef"=w65:refnum<vi>, "ItemTag"=w64:string)  [unwired: 1 in]
            n136 = call "NI_USB6001_Controls_UserMenu.vi"("ItemTag"=w64, "Control Ref"=w65, "error in (no error)"=w67, "VI Server Cluster"=w68) -> ("error out"=w66:errorcluster)  [unwired: 7 in]
          }
          event "AI.Physical.Channel", "AI.Sample.Mode", "AI.TerminalConfiguration", "AI.MaxInputLimit", "AI.MinInputLimit", "AI.SampleRate", "AI.Number.Of.Samples", "AI.Measure", "AI.PhysicalChannel.Include", "AI.MultiChannelAcquisition": Shortcut Menu Selection (User) {
            n137 = event-data() -> ("CtlRef"=w70:refnum<vi>, "ItemTag"=w69:string)  [unwired: 1 in]
            n138 = call "NI_USB6001_Controls_UserMenu.vi"("ItemTag"=w69, "Control Ref"=w70, "error in (no error)"=w73, "VI Server Cluster"=w71) -> ("error out"=w72:errorcluster)  [unwired: 7 in]
          }
          event "LastAction.AddToSecuence": Value Change {
            n139 = event-data() -> ()  [unwired: 1 in, 1 out]
            n140 = call "NI_USB6001_UserLastAction_Add_To_Sequence.vi"("error in (no error)"=w76, "VI Server Cluster"=w75) -> ("error out"=w74:errorcluster)  [unwired: 9 in]
          }
          event "AO.Output", "AO.Physical.Channel", "AO.MinVoltage", "AO.MaxVoltage", "AO.Sample.Clock.Source", "AO.SampleRate", "AO.NumberOfSamples", "AO.GenerationMode", "AO.SinewaveFrequency", "AO.OutputVoltage", "AO.SampleMode", "AO.Update": Value Change {
            n141 = event-data() -> ("CtlRef"=w81:refnum<vi>)  [unwired: 1 in]
            n142 = call "NI_USB6001_Register_User_Last_Action_Analog.vi"("Control in"=w81, "error in (no error)"=w83, "VI Server Cluster"=w82) -> ("error out"=w80:errorcluster, "VI Server Cluster.DUP"=w79:T3)  [unwired: 7 in]
            n143 = call "NI_USB6001_AO_Configuration_Set_Get.vi"("SynchRefs.Set/Get"=SynchRefs_SetGet."Set", "error in (no error)"=w80, "VI Server Cluster"=w79) -> ("error out"=w78:errorcluster)  [unwired: 6 in, 2 out]
          }
          event "DI.Line", "DI.Line.Update", "DI.Port", "DI.Port.Lines.0:7", "DI.Port.Update": Value Change {
            n144 = event-data() -> ("CtlRef"=w84:refnum<vi>)  [unwired: 1 in]
            n145 = call "NI_USB6001_Register_User_Last_Action_Digital.vi"("CtlRef"=w84, "error in (no error)"=w87, "VI Server Cluster"=w86) -> ("error out"=w85:errorcluster)  [unwired: 8 in]
          }
          event "DO.Line.Update", "DO.Line", "DO.Port", "DO.Port.Lines.7:0", "DO.Port.Update", "DO.Line.State": Value Change {
            n146 = event-data() -> ("CtlRef"=w88:refnum<vi>)  [unwired: 1 in]
            n147 = call "NI_USB6001_Register_User_Last_Action_Analog.vi"("Control in"=w88, "error in (no error)"=w91, "VI Server Cluster"=w89) -> ("error out"=w90:errorcluster)  [unwired: 7 in, 1 out]
          }
          event "Cntr.In.Channel", "Cntr.In.Input.Terminal", "Cntr.In.ActiveEdge", "Cntr.In.Sample.Clock.Source", "Cntr.In.IntegrationTime", "Cntr.In.Start": Value Change {
            n148 = event-data() -> ("CtlRef"=w92:refnum<vi>)  [unwired: 1 in]
            n149 = call "NI_USB6001_Register_User_Last_Action_Analog.vi"("Control in"=w92, "error in (no error)"=w95, "VI Server Cluster"=w93) -> ("error out"=w94:errorcluster)  [unwired: 7 in, 1 out]
          }
        }
        n150 = call "NI_USB6001_Accessor_EXIT_Ref.vi"() -> ("EXIT"=w39:refnum<notifier>)  [unwired: 6 in]
        n151 = call "Merge Errors II.vi"("error in 2 (no error)"=w33, "error in 1 (no error)"=w35) -> ("error out.DUP"=w34:errorcluster)  [unwired: 4 in, 1 out]
        n152 = call "StopOnErrorOrCommand.vi"("STOP"=w39, "error in (no error)"=w34) -> ("error out"=w41:errorcluster, "STOP"=w40:bool)  [unwired: 8 in]
      }
      n153 = call "NI_USB6001_DAQmx_AI_Measure.vi"("error in (no error)"=w23, "VI Server Cluster"=w24) -> ("error out"=w27:errorcluster)  [unwired: 9 in]
      n154 = call "NI_USB-6001_AO_Main.vi"("error in (no error)"=w23, "VI Server Cluster"=w24) -> ("error out"=w25:errorcluster)  [unwired: 9 in]
      n155 = call "NI_USB-6001_DAQmx_Counter_IN.vi"("error in (no error)"=w23, "VI Server Cluster"=w24) -> ("error out"=w26:errorcluster)  [unwired: 9 in]
      n156 = call "NI_USB6001_Exeecute_Instructionss_Processor.vi"("error in (no error)"=w23, "VI Server.RefsCluster"=w24) -> ("error out"=w22:errorcluster)  [unwired: 9 in]
      n157 = Build Array(w22, w26, w25, w27, w31) -> (w28:errorcluster[])
      n158 = call "Merge Errors II.vi"("error array in"=w28, "error in 1 (no error)"=w30) -> ("error out.DUP"=w29:errorcluster)  [unwired: 4 in, 1 out]
    }
    frame Error {
    }
  }
  n159 = call-poly "VI Server_GetControl_Value_Ref.vi"("DataType"=tag "" ("DAQmx.Device"), "Control.Label"="DAQmx.Device", "error in"=w12, "SingleInstance"=TRUE, "VI Server.RefsCluster"=w10) -> ("error out"=w15:errorcluster, "Value"=w16:tag, "VI Server.RefsCluster.DUP"=w11:T3)  [unwired: 3 in, 1 out]
  n160 = call <vilib>:"DAQmx Reset Device.vi"("device in"=w16, "error in"=w15) -> ("error out"=w5:errorcluster)  [unwired: 13 in]
  n161 = call "Error 200088_DAQmx_Invalid Task.vi"("DisplayErrorMessage"=FALSE, "error in"=w5) -> ("error out"=w4:errorcluster)  [unwired: 12 in, 1 out]
  n162 = call "VI Server_CloseRefs.vi"("error in"=w4, "VI Server.RefsCluster"=w11) -> ("error out"=w18:errorcluster)  [unwired: 9 in]
  n163 = call "NI_USB6001_Synch_CLOSE.vi"("error in"=w18) -> ("error out"=w8:errorcluster)  [unwired: 10 in]
  n164 = Current VI's Path() -> (path=w6:path)
  n165 = call "Close Window If in EXE mode.vi"("TopLevelVI Path"=w6, "error in"=w8) -> ("error out"=→"error out":errorcluster)  [unwired: 9 in]
